vi "LaunchBall.vi"(8 "error in (no error)":errorcluster) -> (0 "error out":errorcluster)   [LabVIEW 2013]
uses:
  <vilib>/Rock Robotics/WPI/CAN/Jaguar/SubVIs/WPI_CANJaguar_StatusSelect.ctl
  Robot Global Data.vi
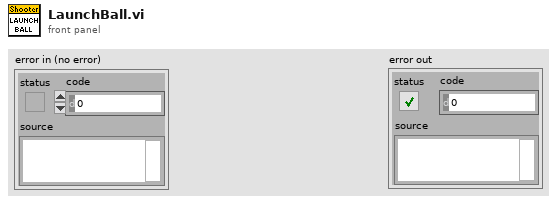
[diagram p1: front panel]
types:
  T1 = typedef "WPI_CANJaguar_StatusSelect.ctl" = enum16{"Output Percent VBus", "Output Voltage", "Bus Voltage", "Current", "Temperature", "Position", "Speed", "Limit Switches", "Faults", "Fault Counters", "Power Cycle"}
  T2 = typedef "WPI_MotorControlDeviceRef.ctl" = cluster{"DeviceStatus":errorcluster, "Type":enum16{"PWM", "CAN"}, "PWM":cluster{"Digital Module":T3, "PWM Channel":T4, "DeadBand":T5}, "CAN":cluster{"Device Number":u8, "Control Mode":T6, "Semaphore":T7, "Max Vout":dbl}, "Invert":bool, "TransformRef":T8, "InvTransformRef":T8}
  T3 = typedef "FPGA_TypedefDigitalModule.ctl" = enum16{"Digital Module 1", "Digital Module 2"}
  T4 = typedef "FPGA_DIOPWMChannel.ctl" = enum8{"PWM 1", "PWM 2", "PWM 3", "PWM 4", "PWM 5", "PWM 6", "PWM 7", "PWM 8", "PWM 9", "PWM 10", "Invalid"}
  T5 = typedef "WPI_PWMDeadband.ctl" = cluster{"Name":string, "maxPositivePwm":i32, "minPositivePwm":i32, "centerPwm":i32, "maxNegativePwm":i32, "minNegativePwm":i32, "angularRange":u16}
  T6 = typedef "WPI_CANJaguar_ControlMode.ctl" = enum8{"Percent VBus", "Current", "Speed", "Position", "Voltage"}
  T7 = typedef "Semaphore RefNum" = refnum<k1>
  T8 = typedef "WPI_PWMTransform_ConPane.ctl" = refnum<vi>
  T9 = typedef "WPI_CANJaguar_Status.ctl" = cluster{"Output Percent VBus":dbl, "Output Voltage":dbl, "Bus Voltage":dbl, "Current":dbl, "Temperature":dbl, "Position":dbl, "Speed":dbl, "Limits":cluster{"Forward Limit":bool, "Reverse Limit":bool, "Forward Soft Limit":bool, "Reverse Soft Limit":bool, "Sticky Forward Limit":bool, "Sticky Reverse Limit":bool, "Sticky Forward Soft Limit":bool, "Sticky Reverse Soft Limit":bool}, "Faults":cluster{"Current Fault":bool, "Temperature Fault":bool, "Bus Voltage Fault":bool, "Gate Driver Fault":bool, "Comm Fault":bool}, "Fault Counters":cluster{"Current Faults":u8, "Temperature Faults":u8, "Bus Voltage Faults":u8, "Gate Driver Faults":u8, "Comm Faults":u8, "CAN Status":u8, "CAN RX Errors":u8, "CAN TX Errors":u8}, "Power Cycle":bool}
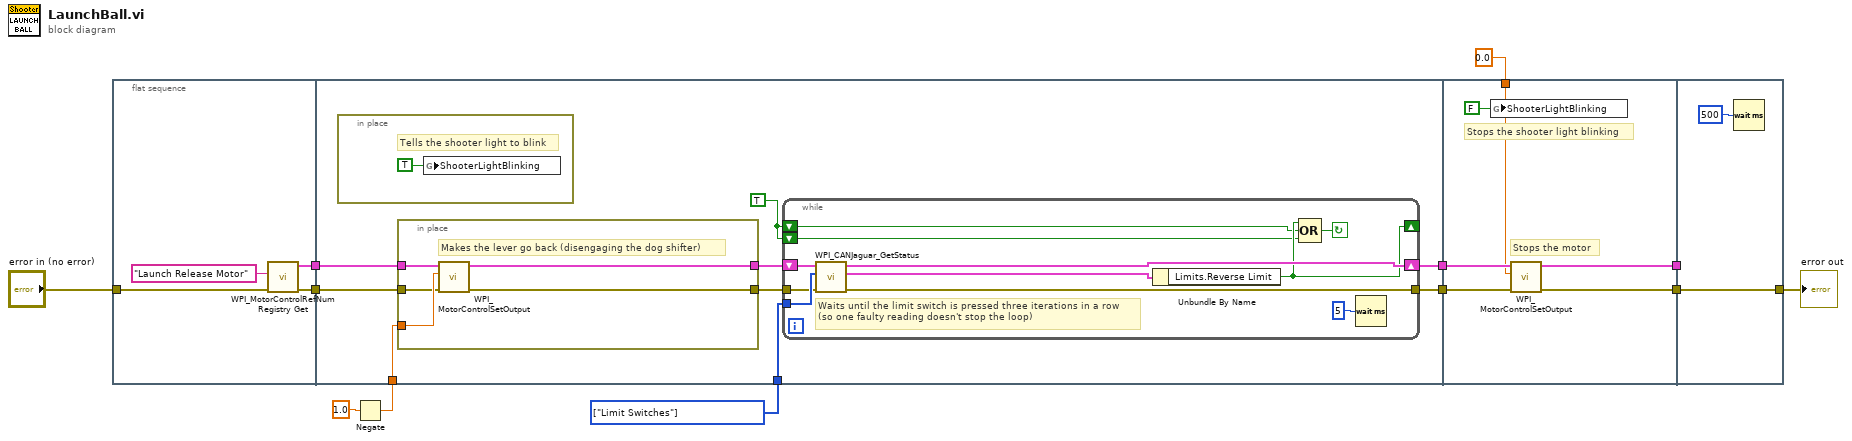
[diagram p0: block diagram]
diagram:
  w7 = T1[] [enum."Limit Switches"] items=["Output Percent VBus", "Output Voltage", "Bus Voltage", "Current", "Temperature", "Position", "Speed", "Limit Switches", "Faults", "Fault Counters", "Power Cycle"] ("Status Select")
  n1 = flat-sequence {
    tunnel: "error in (no error)" -> [w16]
    tunnel: [w14] -> w12
    tunnel: [w13] -> w11
    tunnel: w12 -> [w21]
    tunnel: w11 -> [w20]
    tunnel: [w24] -> w10
    tunnel: [w25] -> w9
    tunnel: w7 -> [w23]
    tunnel: w4 -> [w22]
    tunnel: [w48] -> w6
    tunnel: [w47] -> w5
    tunnel: w9 -> [w45]
    tunnel: w10 -> [w46]
    tunnel: 0.0 ("Output") -> [w44]
    tunnel: w6 -> [_]
    tunnel: w5 -> [w49]
    tunnel: [w49] -> w1
    frame #0 {
      n2 = call <vilib>:"WPI_MotorControlRefNum Registry Get.vi"("error in (no error)"=w16, "refnum name"="Launch Release Motor") -> ("error out"=w13:errorcluster, "MotorControlDevRef"=w14:T2)  [unwired: 8 in]
    }
    frame #1 {
      w17 = TRUE
      n3 = in-place {
        # "Tells the shooter light to blink"
        n4 = global write "Robot Global Data.vi" "ShooterLightBlinking"(TRUE ("ShooterLightBlinking")) -> ()
      }
      n5 = in-place {
        in-place-border: w22 -> [w42]
        in-place-border: w21 -> [w41]
        in-place-border: w20 -> [w40]
        in-place-border: [w39] -> w19
        in-place-border: [w38] -> w18
        # "Makes the lever go back (disengaging the dog shifter)"
        n6 = call <vilib>:"WPI_MotorControlSetOutput.vi"("error in (no error)"=w40, "Output"=w42, "MotorControlDevRef"=w41) -> ("error out"=w38:errorcluster, "MotorControlDevRef"=w39:T2)  [unwired: 6 in, 1 out]
      }
      n7 = while {
        shift-right: [w34] -> w24
        shift-left: w19 -> [w32]
        tunnel: w23 -> [w33]
        tunnel: w18 -> [w31]
        tunnel: [w30] -> w25
        shift-right: [w29] -> _
        shift-left: w17 -> [w28]
        shift-left: w17 -> [w27]
        stop <- w26 continue-if-true
        # "Waits until the limit switch is pressed three iterations in a row\n(so one faulty reading doesn't stop the loop)"
        n8 = call <vilib>:"WPI_CANJaguar_GetStatus.vi"("error in (no error)"=w31, "Status Select"=w33, "CAN Jaguar Ref"=w32) -> ("error out"=w30:errorcluster, "Status"=w36:T9, "CAN Jaguar Ref Out"=w34:T2)  [unwired: 6 in]
        n9 = Unbundle By Name(w36) -> ("Limits.Reverse Limit"=w29:bool)
        n10 = Compound Arithmetic op=OR(w29, w28, w27) -> (w26:bool)
        n11 = Wait (ms)(milliseconds to wait=u32 5) -> ()  [unwired: 1 out]
      }
    }
    frame #2 {
      # "Stops the motor"
      # "Stops the shooter light blinking"
      n12 = global write "Robot Global Data.vi" "ShooterLightBlinking"(FALSE) -> ()
      n13 = call <vilib>:"WPI_MotorControlSetOutput.vi"("error in (no error)"=w45, "Output"=w44, "MotorControlDevRef"=w46) -> ("error out"=w47:errorcluster, "MotorControlDevRef"=w48:T2)  [unwired: 6 in, 1 out]
    }
    frame #3 {
      n14 = Wait (ms)(milliseconds to wait=u32 500) -> ()  [unwired: 1 out]
    }
  }
  n15 = Negate(x=1.0 ("Output")) -> (-x=w4:dbl)
  "error out" <- w1
